vi "yolo-read-png.vi"() -> ()   [LabVIEW 2017]
uses:
  <vilib>/wsapi/NI_WebServices.lvlib
panel:
  out "string out (base64-encoded)":string
  out "Original image":picture
  in  "path to JPEG file":path=path "E:/UPWORK/darknet/labview-meet-yolo/samples/001.jpg"
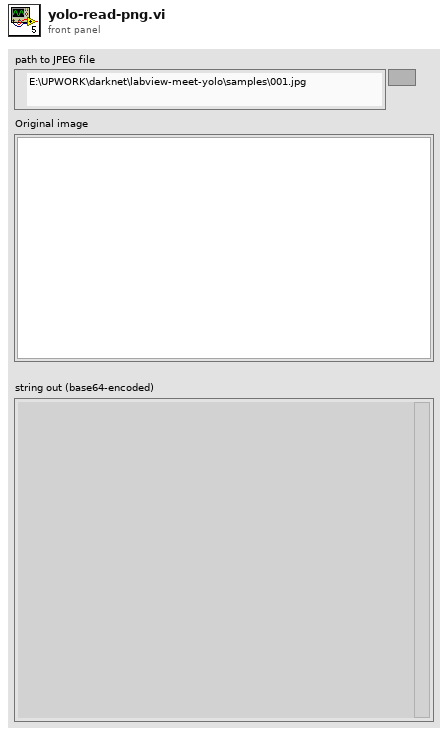
[diagram p1: front panel]
types:
  T1 = typedef "imagedata.ctl" = cluster{"image type":i32, "image depth":i32, "image":u8[], "mask":u8[], "colors":u32[], "Rectangle":cluster{"left":i16, "top":i16, "right":i16, "bottom":i16}}
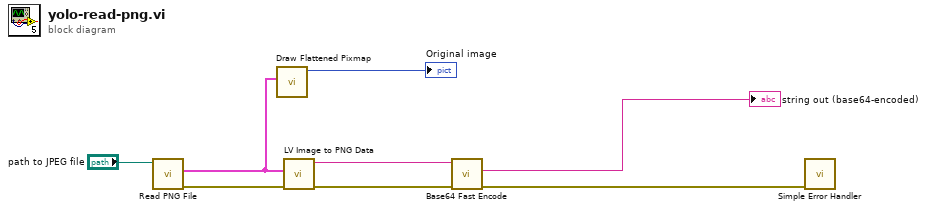
[diagram p0: block diagram]
diagram:
  n1 = call <vilib>:"Read PNG File.vi"("path to PNG file"="path to JPEG file") -> ("error out"=w1:errorcluster, "image data"=w2:T1)  [unwired: 8 in, 1 out]
  n2 = call <vilib>:"Draw Flattened Pixmap.vi"("image data"=w2) -> ("new picture"=→"Original image":picture)  [unwired: 8 in]
  n3 = call <vilib>:"LV Image to PNG Data.vi"("error in (no error)"=w1, "image data"=w2) -> ("error out"=w6:errorcluster, "png data"=w7:string)  [unwired: 8 in]
  n4 = call "Base64 Fast Encode.vi"("error in (no error)"=w6, "string in (not encoded)"=w7) -> ("error out"=w5:errorcluster, "string out (base64-encoded)"=→"string out (base64-encoded)":string)  [unwired: 8 in]
  n5 = call <vilib>:"Simple Error Handler.vi"("error in (no error)"=w5) -> ()  [unwired: 4 in, 5 out]
